vi "Plot_Server_Data.vi"() -> ()   [LabVIEW 2010]
uses:
  Anemometry/Anemometry Sub Vis/Controls/Server_Comms.ctl
  Anemometry/Anemometry Sub Vis/File/Setup_Filetype.ctl
  Anemometry/Anemometry Sub Vis/Globals/Preference_global.vi
panel:
  in  "End from now (min)":dbl format="%.1f"
  in  "Precision":i32=2
  in  "Save 3":bool
  out "Plot 3 Chs":string[](array[string])
  in  "Save 2":bool
  out "Plot 2 Chs":string[](array[string])
  in  "Save 1":bool
  out "Plot 1 Chs":string[](array[string])
  in  "Save plot number":T1(ring)
  in  "Selector 1":i32[](listbox)
  in  "Search 1":string
  in  "Search 2":string
  in  "Search 3":string
  out "Last Updated":string
  out "Plot 3":cluster{"Times":dbl[], "Output array":dbl[]}[](graph)
  in  "Selector 3":i32[](listbox)
  out "Plot 2":cluster{"Times":dbl[], "Output array":dbl[]}[](graph)
  in  "Selector 2":i32[](listbox)
  in  "stop":bool
  in  "Mode":T2(ring)
  out "Plot 1":cluster{dbl[], "Output array":dbl[]}[](graph)
  in  "History (min)":dbl format="%.1f"
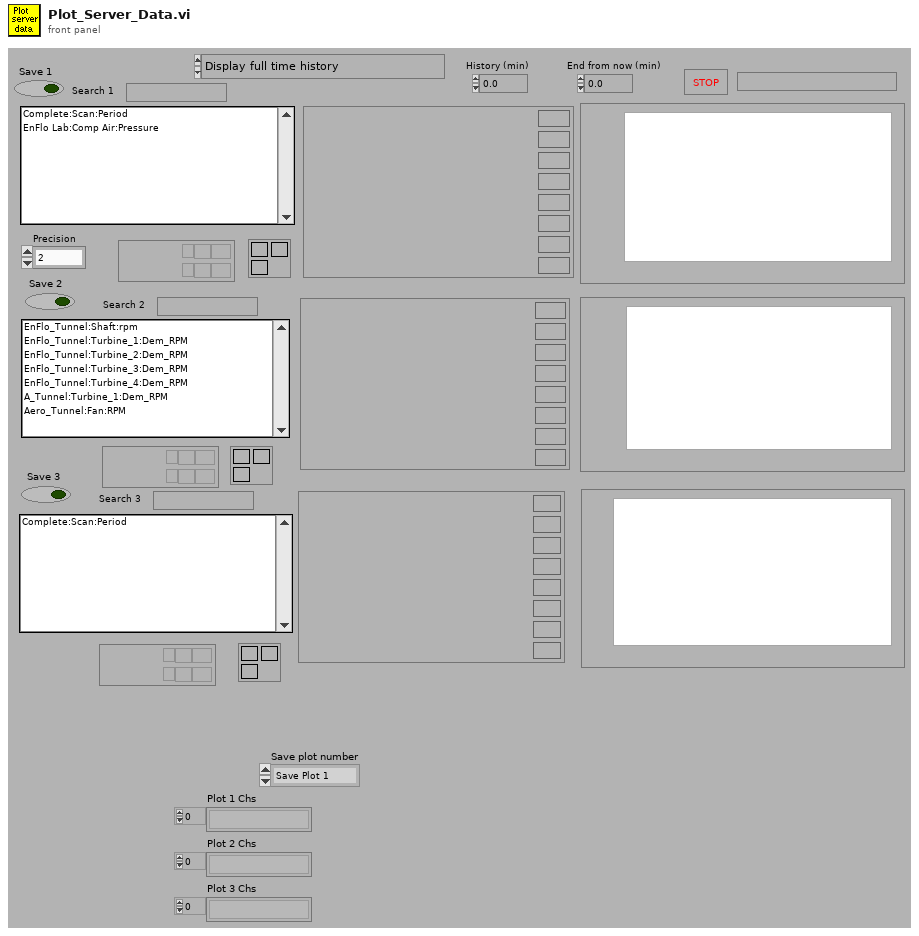
[diagram p1: front panel]
types:
  T1 = enum16{"Save Plot 1", "Save Plot 2", "Save Plot 3"}
  T2 = enum16{"Display full time history", "Display data over specified period"}
  T3 = typedef "Server_Comms.ctl" = enum16{"Server Link Healthy", "Do Not Link To Server"}
  T4 = typedef "Setup_Filetype.ctl" = enum16{"Measurement Setups", "Calibration Setups", "General", "Results File Plotter Setups", "Speed Calib Tweaks"}
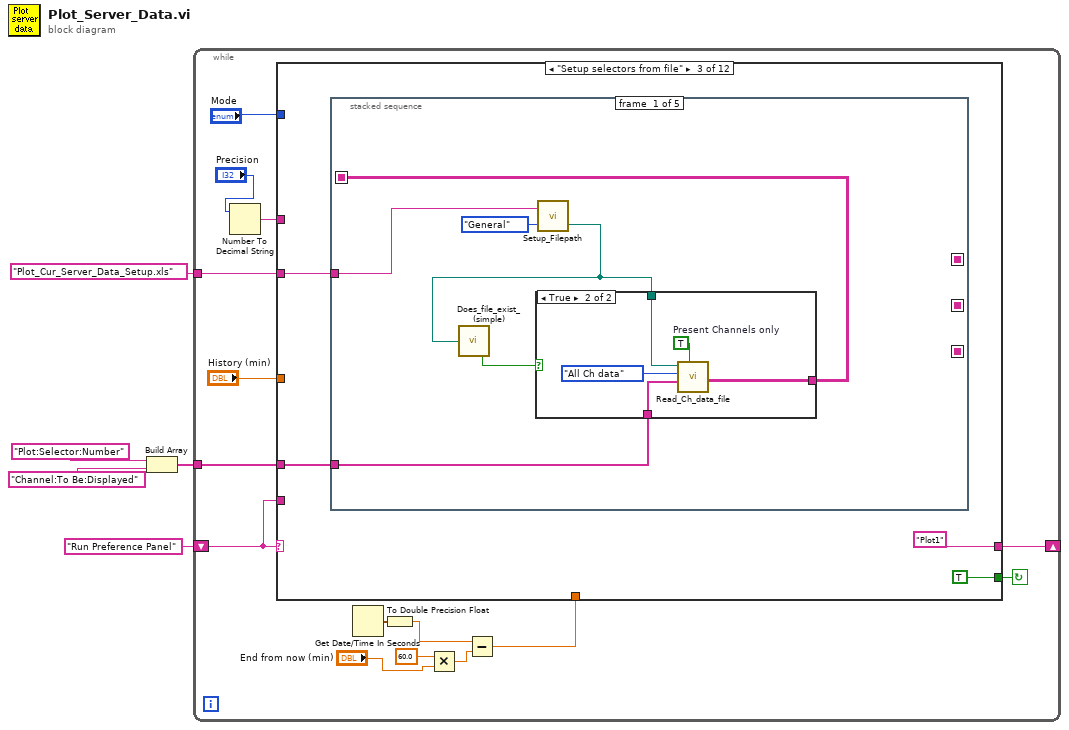
[diagram p0: block diagram]
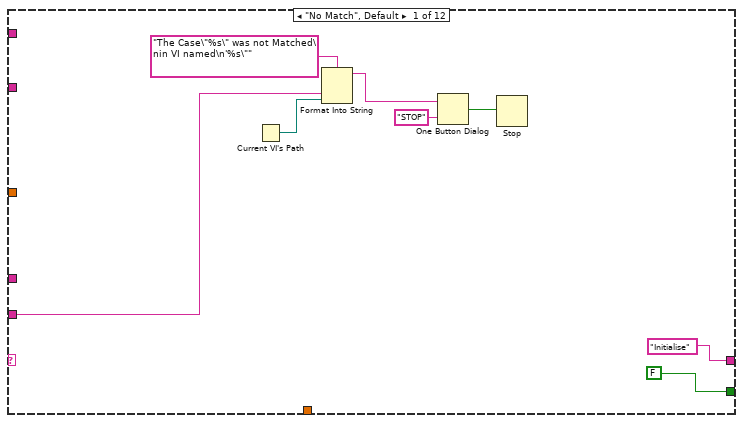
[diagram p2: hidden frame]
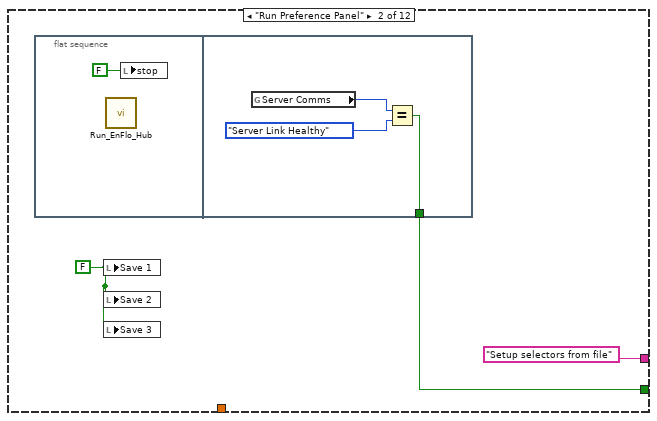
[diagram p3: hidden frame]
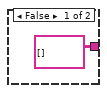
[diagram p4: hidden frame]
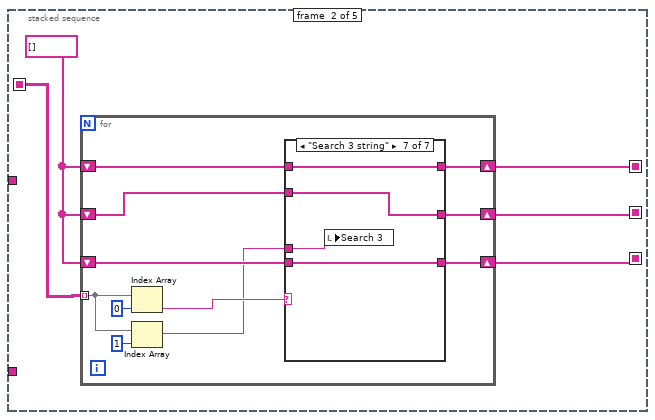
[diagram p5: hidden frame]
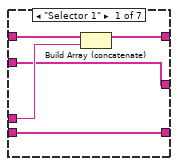
[diagram p6: hidden frame]
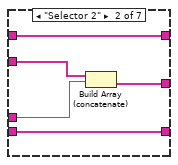
[diagram p7: hidden frame]
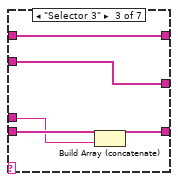
[diagram p8: hidden frame]
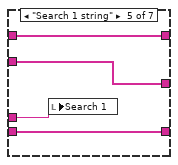
[diagram p10: hidden frame]
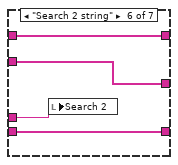
[diagram p11: hidden frame]
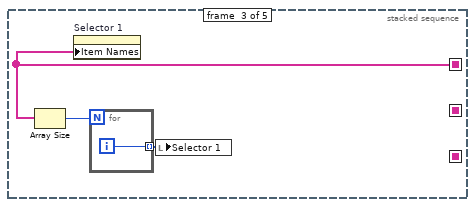
[diagram p12: hidden frame]
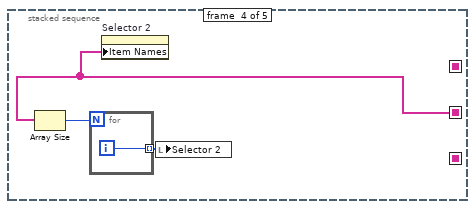
[diagram p13: hidden frame]
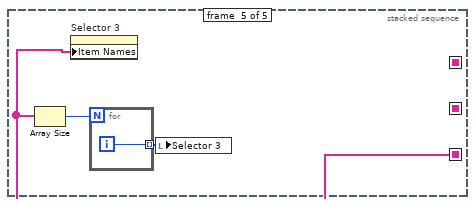
[diagram p14: hidden frame]
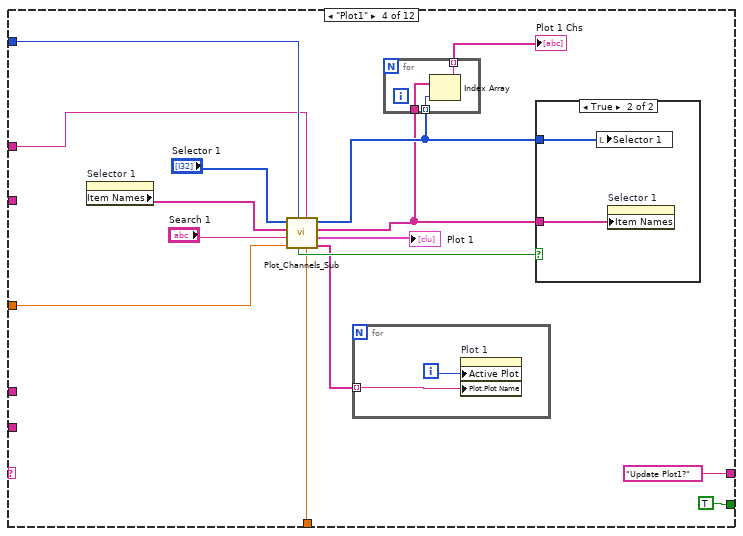
[diagram p15: hidden frame]
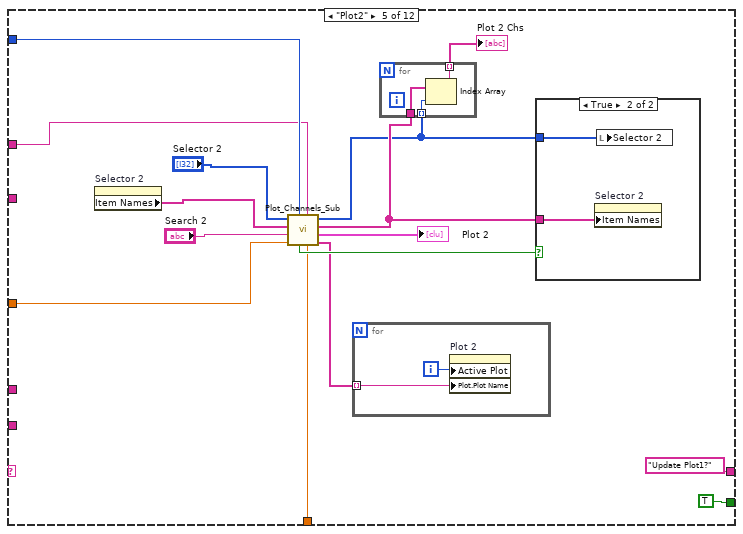
[diagram p17: hidden frame]
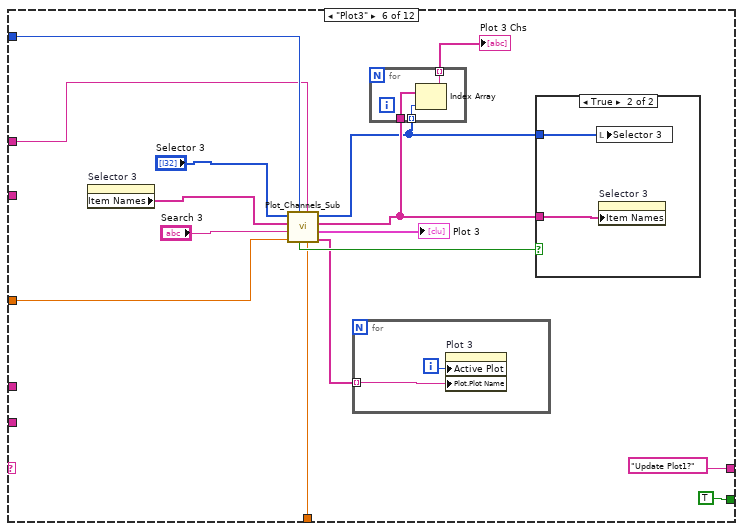
[diagram p19: hidden frame]
diagram:
  n1 = Build Array("Plot:Selector:Number", "Channel:To Be:Displayed") -> (w2:string[])
  n2 = while {
    shift-left: "Run Preference Panel" -> [w18]
    shift-right: [w19] -> _
    tunnel: w2 -> [w15]
    tunnel: "Plot_Cur_Server_Data_Setup.xls" -> [w14]
    stop <- w20 continue-if-true
    n3 = Number To Decimal String(number="Precision") -> (decimal integer string=w12:string)  [unwired: 1 out]
    n4 = Get Date/Time In Seconds() -> (seconds since 1Jan1904=w11:timestamp)
    n5 = To Double Precision Float(number=w11) -> (double precision float=w7:dbl)
    n6 = Multiply(x=60.0, y="End from now (min)") -> (x*y=w8:dbl)
    n7 = Subtract(x=w7, y=w8) -> (x-y=w6:dbl)
    n8 = case shown="\"Setup selectors from file\"" w18 {
      tunnel: [FALSE w30 TRUE TRUE TRUE TRUE TRUE TRUE TRUE TRUE w302 w360] -> w20
      tunnel: ["Initialise" "Setup selectors from file" "Plot1" "Update Plot1?" "Update Plot1?" "Update Plot1?" w177 w198 w218 w250 w303 "Update Plot1?" ("t")] -> w19
      tunnel: w18 -> [w23 _ _ _ _ _ _ _ _ _ _ _]
      tunnel: "Mode" -> [_ _ _ w117 w143 w165 _ _ _ _ _ _]
      tunnel: "History (min)" -> [_ _ _ w116 w142 w164 _ _ _ _ _ _]
      tunnel: w15 -> [_ _ w36 _ _ _ _ _ _ _ _ w364]
      tunnel: w14 -> [_ _ w37 _ _ _ _ _ _ _ _ w363]
      tunnel: w12 -> [_ _ _ w111 w133 w155 _ _ _ _ _ _]
      tunnel: w6 -> [_ _ _ w110 w132 w154 _ _ _ _ _ _]
      frame "No Match", Default {
        n9 = Current VI's Path() -> (path=w22:path)
        n10 = Format Into String(format string="The Case\"%s\" was not Matched\nin VI named\n'%s\"" ("Format String"), w23, w22) -> (resulting string=w26:string)  [unwired: 2 in, 1 out]
        n11 = One Button Dialog(message=w26, button name ("OK")="STOP") -> (true=w24:bool)
        n12 = Stop(stop? (T)=w24) -> ()
      }
      frame "Run Preference Panel" {
        w29 = FALSE ("Save 1")
        n13 = flat-sequence {
          tunnel: [w33] -> w30
          frame #0 {
            n14 = call "Run_EnFlo_Hub.vi"() -> ()  [unwired: 8 out]
            n15 = local write "stop"(FALSE ("stop")) -> ()
          }
          frame #1 {
            n16 = global read "Preference_global.vi" "Server Comms"() -> (w34:T3)
            n17 = Equal?(x=w34, y=Server_Comms."Server Link Healthy" ("Server Comms")) -> (x = y?=w33:bool)
          }
        }
        n18 = local write "Save 1"(w29) -> ()
        n19 = local write "Save 2"(w29) -> ()
        n20 = local write "Save 3"(w29) -> ()
      }
      frame "Setup selectors from file" {
        n21 = stacked-sequence {
          seq-local: [w43 _ _ _ _] -> [_ w56 _ _ _]
          seq-local: [_ w54 _ _ _] -> [_ _ w100 _ _]
          seq-local: [_ w52 _ _ _] -> [_ _ _ w102 _]
          seq-local: [_ w53 _ _ _] -> [_ _ _ _ w106]
          tunnel: w37 -> [w42 _ _ _ _]
          tunnel: w36 -> [w44 _ _ _ _]
          frame #0 {
            n22 = call "Setup_Filepath.vi"("Setup File Type"=Setup_Filetype."General", "Filename in"=w42) -> ("Filename Out"=w41:path)  [unwired: 1 out]
            n23 = call "Does_file_exist_(simple).vi"("Pathname"=w41) -> ("exists?"=w45:bool)
            n24 = case shown="True" w45 {
              tunnel: w41 -> [_ w51]
              tunnel: w44 -> [_ w50]
              tunnel: [string[][] [] ("Channel Values") w47] -> w43
              frame False {
              }
              frame True {
                w49 = TRUE  # Present Channels only
                n25 = call "Read_Ch_data_file.vi"("Present Channels only"=w49, "Present Channels"=w50, "Output"=enum16{"All Ch data", "The last few rows"}."All Ch data", "Filename"=w51) -> ("Channel Values"=w47:string[][])  [unwired: 1 in, 4 out]
              }
            }
          }
          frame #1 {
            w55 = string[] []
            n26 = for {
              shift-right: [w62] -> w54
              shift-left: w55 -> [w63]
              tunnel: w56 -> [w64] mode=indexing
              shift-right: [w60] -> w52
              shift-left: w55 -> [w61]
              shift-right: [w58] -> w53
              shift-left: w55 -> [w59]
              n27 = Index Array(array=w64, index=0 ("Index")) -> (element=w66:string)
              n28 = Index Array(array=w64, index=1 ("Index")) -> (element=w57:string)
              n29 = case shown="\"Search 3 string\"" w66 {
                tunnel: w63 -> [w72 w77 w78 w84 w88 w92 w96]
                tunnel: [w71 w77 w78 w84 w88 w92 w96] -> w62
                tunnel: w57 -> [w70 w74 w80 _ w86 w90 w94]
                tunnel: w61 -> [w69 w75 w79 w85 w89 w93 w97]
                tunnel: [w69 w73 w79 w85 w89 w93 w97] -> w60
                tunnel: w59 -> [w68 w76 w82 w83 w87 w91 w95]
                tunnel: [w68 w76 w81 w83 w87 w91 w95] -> w58
                frame "Selector 1" {
                  n30 = Build Array (concatenate)(w72, w70) -> (w71:string[])
                }
                frame "Selector 2" {
                  n31 = Build Array (concatenate)(w75, w74) -> (w73:string[])
                }
                frame "Selector 3" {
                  n32 = Build Array (concatenate)(w82, w80) -> (w81:string[])
                }
                frame "No Match", Default {
                }
                frame "Search 1 string" {
                  n33 = local write "Search 1"(w86) -> ()
                }
                frame "Search 2 string" {
                  n34 = local write "Search 2"(w90) -> ()
                }
                frame "Search 3 string" {
                  n35 = local write "Search 3"(w94) -> ()
                }
              }
            }
          }
          frame #2 {
            n36 = Array Size(array=w100) -> (size(s)=w99:i32)
            n37 = property on="Selector 1" class="LstBox (strict)"("Item Names"=w100) -> ()  [unwired: 2 in, 2 out]
            n38 = for {
              N: w99 -> [_]
              tunnel: [w101] -> w98 mode=indexing
              i -> [w101]
            }
            n39 = local write "Selector 1"(w98) -> ()
          }
          frame #3 {
            n40 = Array Size(array=w102) -> (size(s)=w104:i32)
            n41 = for {
              N: w104 -> [_]
              tunnel: [w105] -> w103 mode=indexing
              i -> [w105]
            }
            n42 = property on="Selector 2" class="LstBox (strict)"("Item Names"=w102) -> ()  [unwired: 2 in, 2 out]
            n43 = local write "Selector 2"(w103) -> ()
          }
          frame #4 {
            n44 = Array Size(array=w106) -> (size(s)=w108:i32)
            n45 = property on="Selector 3" class="LstBox (strict)"("Item Names"=w106) -> ()  [unwired: 2 in, 2 out]
            n46 = for {
              N: w108 -> [_]
              tunnel: [w109] -> w107 mode=indexing
              i -> [w109]
            }
            n47 = local write "Selector 3"(w107) -> ()
          }
        }
      }
      frame "Plot1" {
        n48 = property on="Selector 1" class="LstBox (strict)"() -> ("Item Names"=w119:string[])  [unwired: 2 in, 2 out]
        n49 = call "Plot_Channels_Sub.vi"("End Time"=w110, "precision"=w111, "Mode"=w117, "History (min)"=w116, "Search String"="Search 1", "Selector List In"=w119, "Selector array In"="Selector 1") -> ("Plot Legend"=w115:string[], "Plot"=→"Plot 1":cluster{"Times":dbl[], "Output array":dbl[]}[], "Selector List Out"=w113:string[], "Selector array Out"=w114:i32[], "Selector Changed?"=w121:bool)
        n50 = for {
          tunnel: w115 -> [w128] mode=indexing
          i -> [w129]
          n51 = property on="Plot 1" class="XYGraph (strict)"("Active Plot"=w129, "Plot.Plot Name"=w128) -> ()  [unwired: 2 in, 2 out]
        }
        n52 = for {
          tunnel: w114 -> [w127] mode=indexing
          tunnel: w113 -> [w126]
          tunnel: [w125] -> w112 mode=indexing
          n53 = Index Array(array=w126, index=w127) -> (element=w125:string)
        }
        "Plot 1 Chs" <- w112
        n54 = case shown="True" w121 {
          tunnel: w113 -> [_ w131]
          tunnel: w114 -> [_ w130]
          frame False {
          }
          frame True {
            n55 = local write "Selector 1"(w130) -> ()
            n56 = property on="Selector 1" class="LstBox (strict)"("Item Names"=w131) -> ()  [unwired: 2 in, 2 out]
          }
        }
      }
      frame "Plot2" {
        n57 = property on="Selector 2" class="LstBox (strict)"() -> ("Item Names"=w138:string[])  [unwired: 2 in, 2 out]
        n58 = call "Plot_Channels_Sub.vi"("End Time"=w132, "precision"=w133, "Mode"=w143, "History (min)"=w142, "Search String"="Search 2", "Selector List In"=w138, "Selector array In"="Selector 2") -> ("Plot Legend"=w137:string[], "Plot"=→"Plot 2":cluster{"Times":dbl[], "Output array":dbl[]}[], "Selector List Out"=w136:string[], "Selector array Out"=w135:i32[], "Selector Changed?"=w144:bool)
        n59 = for {
          tunnel: w137 -> [w150] mode=indexing
          i -> [w151]
          n60 = property on="Plot 2" class="XYGraph (strict)"("Active Plot"=w151, "Plot.Plot Name"=w150) -> ()  [unwired: 2 in, 2 out]
        }
        n61 = for {
          tunnel: w135 -> [w149] mode=indexing
          tunnel: w136 -> [w148]
          tunnel: [w147] -> w134 mode=indexing
          n62 = Index Array(array=w148, index=w149) -> (element=w147:string)
        }
        "Plot 2 Chs" <- w134
        n63 = case shown="True" w144 {
          tunnel: w136 -> [_ w152]
          tunnel: w135 -> [_ w153]
          frame False {
          }
          frame True {
            n64 = property on="Selector 2" class="LstBox (strict)"("Item Names"=w152) -> ()  [unwired: 2 in, 2 out]
            n65 = local write "Selector 2"(w153) -> ()
          }
        }
      }
      frame "Plot3" {
        n66 = property on="Selector 3" class="LstBox (strict)"() -> ("Item Names"=w160:string[])  [unwired: 2 in, 2 out]
        n67 = call "Plot_Channels_Sub.vi"("End Time"=w154, "precision"=w155, "Mode"=w165, "History (min)"=w164, "Search String"="Search 3", "Selector List In"=w160, "Selector array In"="Selector 3") -> ("Plot Legend"=w159:string[], "Plot"=→"Plot 3":cluster{"Times":dbl[], "Output array":dbl[]}[], "Selector List Out"=w158:string[], "Selector array Out"=w157:i32[], "Selector Changed?"=w166:bool)
        n68 = for {
          tunnel: w159 -> [w172] mode=indexing
          i -> [w173]
          n69 = property on="Plot 3" class="XYGraph (strict)"("Active Plot"=w173, "Plot.Plot Name"=w172) -> ()  [unwired: 2 in, 2 out]
        }
        n70 = for {
          tunnel: w157 -> [w171] mode=indexing
          tunnel: w158 -> [w170]
          tunnel: [w169] -> w156 mode=indexing
          n71 = Index Array(array=w170, index=w171) -> (element=w169:string)
        }
        "Plot 3 Chs" <- w156
        n72 = case shown="True" w166 {
          tunnel: w158 -> [_ w174]
          tunnel: w157 -> [_ w175]
          frame False {
          }
          frame True {
            n73 = local write "Selector 3"(w175) -> ()
            n74 = property on="Selector 3" class="LstBox (strict)"("Item Names"=w174) -> ()  [unwired: 2 in, 2 out]
          }
        }
      }
      frame "Update Plot1?" {
        n75 = while {
          shift-right: [w195] -> w184
          shift-left: _ -> [w192]
          shift-right: [w194] -> w186
          shift-left: _ -> [w193]
          tunnel: [w193] -> w185
          tunnel: [w192] -> w183
          stop <- FALSE continue-if-true
          n76 = local read "Selector 1"() -> (w195:i32[])
          n77 = local read "Search 1"() -> (w194:string)
        }
        n78 = case shown="False" "Save 1" {
          tunnel: ["Update Plot2?" "Save Plot" ("t")] -> w176
          frame False {
          }
          frame True {
            n79 = local write "Save plot number"(T1."Save Plot 1" ("Save plot number")) -> ()
          }
        }
        n80 = Equal?(x=w184, y=w183) -> (x = y?=w181:bool)
        n81 = Equal?(x=w185, y=w186) -> (x = y?=w182:bool)
        n82 = And(x=w181, y=w182) -> (x .and. y?=w180:bool)
        n83 = Select(t=w176, s=w180, f="Plot1") -> (s? t:f=w177:string)
      }
      frame "Update Plot2?" {
        n84 = while {
          shift-right: [w215] -> w204
          shift-left: _ -> [w212]
          shift-right: [w214] -> w206
          shift-left: _ -> [w213]
          tunnel: [w213] -> w205
          tunnel: [w212] -> w203
          stop <- FALSE continue-if-true
          n85 = local read "Selector 2"() -> (w215:i32[])
          n86 = local read "Search 2"() -> (w214:string)
        }
        n87 = case shown="False" "Save 2" {
          tunnel: ["Update Plot3?" "Save Plot" ("t")] -> w196
          frame False {
          }
          frame True {
            n88 = local write "Save plot number"(T1."Save Plot 2" ("Save plot number")) -> ()
          }
        }
        n89 = Equal?(x=w204, y=w203) -> (x = y?=w201:bool)
        n90 = Equal?(x=w205, y=w206) -> (x = y?=w202:bool)
        n91 = And(x=w201, y=w202) -> (x .and. y?=w200:bool)
        n92 = Select(t=w196, s=w200, f="Plot2") -> (s? t:f=w198:string)
      }
      frame "Update Plot3?" {
        n93 = while {
          shift-right: [w235] -> w224
          shift-left: _ -> [w232]
          shift-right: [w234] -> w226
          shift-left: _ -> [w233]
          tunnel: [w233] -> w225
          tunnel: [w232] -> w223
          stop <- FALSE continue-if-true
          n94 = local read "Selector 3"() -> (w235:i32[])
          n95 = local read "Search 3"() -> (w234:string)
        }
        n96 = case shown="False" "Save 3" {
          tunnel: ["What to do next?" "Save Plot" ("t")] -> w216
          frame False {
          }
          frame True {
            n97 = local write "Save plot number"(T1."Save Plot 3" ("Save plot number")) -> ()
          }
        }
        n98 = Equal?(x=w224, y=w223) -> (x = y?=w221:bool)
        n99 = Equal?(x=w225, y=w226) -> (x = y?=w222:bool)
        n100 = And(x=w221, y=w222) -> (x .and. y?=w220:bool)
        n101 = Select(t=w216, s=w220, f="Plot3") -> (s? t:f=w218:string)
      }
      frame "What to do next?" {
        n102 = Wait (ms)(milliseconds to wait=u32 300) -> ()  [unwired: 1 out]
        n103 = while {
          shift-right: [w266] -> _
          shift-left: _ -> [w265]
          shift-right: [w264] -> _
          shift-left: _ -> [w263]
          shift-right: [w256] -> _
          shift-left: _ -> [w255]
          tunnel: [w258] -> w249
          shift-right: [w252] -> w237
          shift-left: _ -> [w253]
          stop <- FALSE continue-if-true
          n104 = local read "History (min)"() -> (w266:dbl)
          n105 = local read "Mode"() -> (w264:T2)
          n106 = Equal?(x=w266, y=w265) -> (x = y?=w262:bool)
          n107 = Equal?(x=w263, y=w264) -> (x = y?=w261:bool)
          n108 = And(x=w262, y=w261) -> (x .and. y?=w260:bool)
          n109 = Select(t=w255, s=w260, f=0) -> (s? t:f=w257:i32)
          n110 = case shown="0, Default" w257 {
            tunnel: ["Plot1" "Plot2" "Plot3" "Update Plot1?" "Update Plot1?" "Update Plot1?" "Update Plot1?"] -> w258
            tunnel: w257 -> [w269 w273 w277 w283 w289 w295 _]
            tunnel: [w268 w272 w276 w282 w288 w294 0] -> w256
            tunnel: w253 -> [w267 w271 w275 w280 w286 w291 w298]
            tunnel: [w267 w271 w275 w279 w285 w292 w297] -> w252
            frame 0, Default {
              n111 = Increment(x=w269) -> (x+1=w268:i32)
            }
            frame 1 {
              n112 = Increment(x=w273) -> (x+1=w272:i32)
            }
            frame 2 {
              n113 = Increment(x=w277) -> (x+1=w276:i32)
            }
            frame 3 {
              n114 = Add(x=w280, y=1) -> (x+y=w279:i32)
              n115 = Increment(x=w283) -> (x+1=w282:i32)
            }
            frame 4 {
              n116 = Add(x=w286, y=1) -> (x+y=w285:i32)
              n117 = Increment(x=w289) -> (x+1=w288:i32)
            }
            frame 5 {
              n118 = Add(x=w291, y=1) -> (x+y=w292:i32)
              n119 = Increment(x=w295) -> (x+1=w294:i32)
            }
            frame 6 {
              n120 = Add(x=w298, y=1) -> (x+y=w297:i32)
            }
          }
        }
        n121 = Get Date/Time String(date format (0)=enum16{"short", "long", "abbreviated"}."abbreviated") -> (date string=w245:string, time string=w246:string)  [unwired: 2 out]
        n122 = Concatenate Strings(w245, " at " ("Substring"), w246) -> (→"Last Updated":string)
        n123 = Quotient & Remainder(x=w237, y=500) -> (x-y*floor(x/y)=w241:i32)  [unwired: 1 out]
        n124 = Equal To 0?(x=w241) -> (x = 0?=w239:bool)
        n125 = Or(x="stop", y=w239) -> (x .or. y?=w238:bool)
        n126 = Select(t="Save Channel Names", s=w238, f=w249) -> (s? t:f=w250:string)
      }
      frame "Save Plot" {
        n127 = stacked-sequence {
          seq-local: [w312 _] -> [_ w338]
          seq-local: [w307 _] -> [_ w340]
          seq-local: [w311 _] -> [_ w339]
          tunnel: ["What to do next?" _] -> w303
          tunnel: [TRUE _] -> w302
          frame #0 {
            n128 = case shown="\"Save Plot 1\"" "Save plot number" {
              tunnel: [w320 w323 w326] -> w317
              tunnel: [w319 w322 w325] -> w312
              frame "Save Plot 1" {
                n129 = local read "Plot 1 Chs"() -> (w319:string[])
                n130 = local write "Save 1"(FALSE ("Save 1")) -> ()
                n131 = local read "Plot 1"() -> (w320:cluster{dbl[], "Output array":dbl[]}[])
              }
              frame "Save Plot 2" {
                n132 = local read "Plot 2 Chs"() -> (w322:string[])
                n133 = local write "Save 2"(FALSE ("Save 1")) -> ()
                n134 = local read "Plot 2"() -> (w323:cluster{"Times":dbl[], "Output array":dbl[]}[])
              }
              frame "Save Plot 3" {
                n135 = local read "Plot 3 Chs"() -> (w325:string[])
                n136 = local write "Save 3"(FALSE ("Save 1")) -> ()
                n137 = local read "Plot 3"() -> (w326:cluster{"Times":dbl[], "Output array":dbl[]}[])
              }
            }
            n138 = Index Array(array=w317, index=0) -> (element=w315:cluster{"Times":dbl[], "Output array":dbl[]})
            n139 = Unbundle(w315) -> ("Times"=w305:dbl[])  [unwired: 1 out]
            n140 = Get Date/Time In Seconds() -> (seconds since 1Jan1904=w309:timestamp)
            n141 = for {
              tunnel: w317 -> [w328] mode=indexing
              tunnel: [w327] -> w311 mode=indexing
              n142 = Unbundle(w328) -> ("Output array"=w327:dbl[])  [unwired: 1 out]
            }
            n143 = To Double Precision Float(number=w309) -> (double precision float=w308:dbl)
            n144 = Multiply(x=w305, y=60.0) -> (x*y=w306:dbl[])
            n145 = Add(x=w308, y=w306) -> (x+y=w307:dbl[])
          }
          frame #1 {
            w333 = FALSE  # append to file? (new file:F)
            n146 = for {
              tunnel: w339 -> [w357]
              tunnel: w340 -> [w351] mode=indexing
              tunnel: [w353] -> w332 mode=indexing
              i -> [w356]
              n147 = Number To Decimal String(number=w351) -> (decimal integer string=w352:string)  [unwired: 1 out]
              n148 = Index Array(array=w357, index (col)=w356) -> (element=w355:dbl[])  [unwired: 1 in]
              n149 = Get Date/Time String(seconds (now)=w351) -> (date string=w350:string, time string=w349:string)  [unwired: 2 out]
              n150 = for {
                tunnel: w355 -> [w359] mode=indexing
                tunnel: [w358] -> w354 mode=indexing
                n151 = call "Number_2_string.vi"("number"=w359) -> ("String"=w358:string)  [unwired: 1 in]
              }
              n152 = Build Array (concatenate)(w350, w349, w352, w354) -> (w353:string[])
            }
            n153 = Build Array (concatenate)("Date::", "Centre:Time:", "Seconds:Since:1st Jan 1904", w338) -> (w331:string[])
            n154 = call "Ch_names_to_rows.vi"("Channel Names"=w331) -> ("3 Row names"=w337:string[][])
            n155 = File Dialog(7:"Please choose file name" ("prompt")) -> (3:w345:path)  [unwired: 1 in, 8 out]
            n156 = Build Array (concatenate)(w337, w332) -> (w335:string[][])
            n157 = Strip Path(path=w345) -> (stripped path=w342:path, name=w344:string)
            n158 = call "Add_filename_suffix.vi"("Filename"=w344, "Suffix to add"=".xls") -> ("Filename out"=w341:string)  [unwired: 3 out]
            n159 = Array To Spreadsheet String(array=w335, 3:"%s" ("format string")) -> (spreadsheet string=w334:string)  [unwired: 1 out]
            n160 = Build Path(base path=w342, name or relative path=w341) -> (appended path=w330:path)
            n161 = call "Write_File_Simple.vi"("append to file? (new file:F)"=w333, "character string"=w334, "file path"=w330) -> ()  [unwired: 2 out]
          }
        }
      }
      frame "Save Channel Names" {
        n162 = stacked-sequence {
          seq-local: [w366 _ _] -> [_ w390 _]
          seq-local: [_ w389 _] -> [_ _ w403]
          tunnel: w364 -> [_ _ w404]
          tunnel: w363 -> [_ _ w401]
          frame #0 {
            n163 = for {
              N: 3 -> [_]
              shift-right: [w370] -> w366
              shift-left: string[][] [] -> [w372]
              i -> [w377]
              n164 = Increment(x=w377) -> (x+1=w374:i32)
              n165 = case shown="2" w374 {
                tunnel: [w384 w385 w387] -> w376
                tunnel: [w383 w386 w388] -> w368
                frame 1, Default {
                  n166 = local read "Selector 1"() -> (w384:i32[])
                  n167 = property on="Selector 1" class="LstBox (strict)"() -> ("Item Names"=w383:string[])  [unwired: 2 in, 2 out]
                }
                frame 2 {
                  n168 = property on="Selector 2" class="LstBox (strict)"() -> ("Item Names"=w386:string[])  [unwired: 2 in, 2 out]
                  n169 = local read "Selector 2"() -> (w385:i32[])
                }
                frame 3 {
                  n170 = local read "Selector 3"() -> (w387:i32[])
                  n171 = property on="Selector 3" class="LstBox (strict)"() -> ("Item Names"=w388:string[])  [unwired: 2 in, 2 out]
                }
              }
              n172 = Format Into String(format string="%d" ("Format String"), initial string="Selector ", w374) -> (resulting string=w371:string)  [unwired: 1 in, 1 out]
              n173 = for {
                tunnel: w376 -> [w382] mode=indexing
                tunnel: w371 -> [w381]
                tunnel: [w379] -> w369 mode=indexing
                tunnel: w368 -> [w378]
                n174 = Index Array(array=w378, index=w382) -> (element=w380:string)
                n175 = Build Array(w381, w380) -> (w379:string[])
              }
              n176 = Build Array (concatenate)(w372, w369) -> (w370:string[][])
            }
          }
          frame #1 {
            n177 = local read "Search 1"() -> (w391:string)
            n178 = local read "Search 2"() -> (w392:string)
            n179 = local read "Search 3"() -> (w393:string)
            n180 = Build Array("Search 1 string" ("element"), w391) -> (w397:string[])
            n181 = Build Array("Search 3 string" ("element"), w393) -> (w399:string[])
            n182 = Build Array("Search 2 string" ("element"), w392) -> (w398:string[])
            n183 = Build Array (concatenate)(w390, w397, w398, w399) -> (w389:string[][])
          }
          frame #2 {
            n184 = call "Setup_Filepath.vi"("Setup File Type"=Setup_Filetype."General", "Filename in"=w401) -> ("Filename Out"=w400:path)  [unwired: 1 out]
            n185 = Array Size(array=w403) -> (size(s)=w407:i32[])
            n186 = Index Array(array=w407, index=1 ("Index")) -> (element=w406:i32)
            n187 = Not Equal To 0?(x=w406) -> (x != 0?=w405:bool)
            n188 = case shown="True" w405 {
              tunnel: w400 -> [w409 w414]
              tunnel: w403 -> [_ w415]
              tunnel: w404 -> [_ w416]
              frame False {
                n189 = Delete(path (use dialog)=w409) -> ()  [unwired: 1 in, 6 out]
              }
              frame True {
                w410 = FALSE  # append to file? (new file:F)
                n190 = call "Ch_names_to_rows.vi"("Channel Names"=w416) -> ("3 Row names"=w417:string[][])
                n191 = Build Array (concatenate)(w417, w415) -> (w412:string[][])
                n192 = Array To Spreadsheet String(array=w412, 3:"%s" ("format string")) -> (spreadsheet string=w411:string)  [unwired: 1 out]
                n193 = call "Write_File_Simple.vi"("append to file? (new file:F)"=w410, "character string"=w411, "file path"=w414) -> ()  [unwired: 2 out]
              }
            }
          }
        }
        n194 = local read "stop"() -> (w361:bool)
        n195 = Not(x=w361) -> (.not. x?=w360:bool)
      }
    }
  }
